vi "Day 15 - HASH.vi"(11 "String":string) -> (3 "HASH":i32)   [LabVIEW 2021]
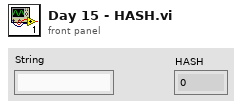
[diagram p1: front panel]
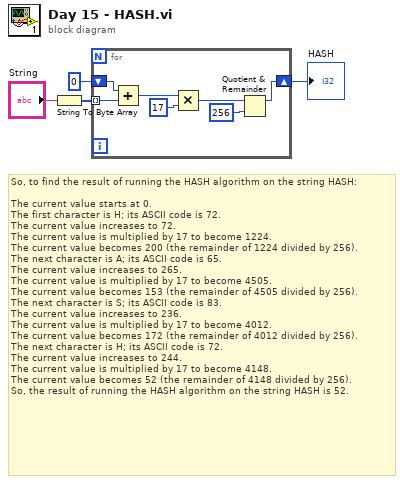
[diagram p0: block diagram]
diagram:
  # "So, to find the result of running the HASH algorithm on the string HASH:\n\nThe current value starts at 0.\nThe first character is H; its ASCII code is 72.\nThe current value increases to 72.\nThe current value is multiplied by 17 to become 1224.\nThe current value becomes 200 (the remainder of 1224 divided by 256).\nThe next character is A; its ASCII code is 65.\nThe current value increases to 265.\nThe current value is multiplied by 17 to become 4505.\nThe current value becomes 153 (the remainder of 4505 divided by 256).\nThe next character is S; its ASCII code is 83.\nThe current value increases to 236.\nThe current value is multiplied by 17 to become 4012.\nThe current value becomes 172 (the remainder of 4012 divided by 256).\nThe next character is H; its ASCII code is 72.\nThe current value increases to 244.\nThe current value is multiplied by 17 to become 4148.\nThe current value becomes 52 (the remainder of 4148 divided by 256).\nSo, the result of running the HASH algorithm on the string HASH is 52."
  n1 = String To Byte Array(string="String") -> (unsigned byte array=w3:u8[])
  n2 = for {
    tunnel: w3 -> [w10] mode=indexing
    shift-right: [w5] -> w1
    shift-left: 0 -> [w11]
    n3 = Add(x=w11, y=w10) -> (x+y=w9:i32)
    n4 = Multiply(x=w9, y=17) -> (x*y=w7:i32)
    n5 = Quotient & Remainder(x=w7, y=256) -> (x-y*floor(x/y)=w5:i32)  [unwired: 1 out]
  }
  "HASH" <- w1
